vi "simx Get Objects.vi"(6 "operationMode":i32, 7 "objectHandles":i32, 8 "error in (no error)":errorcluster, 9 "objectCount":i32, 10 "objectType":i32, 11 "clientID":i32) -> (0 "error out":errorcluster, 1 "objectCount out":i32, 3 "function return":i32, 5 "objectHandles out":i32)   [LabVIEW 2019, in "PXL_V-REP.lvlib"]
doc: "EXTAPI_DLLEXPORT simxInt simxGetObjects(simxInt clientID,simxInt objectType,simxInt* objectCount,simxInt** objectHandles,simxInt operationMode);"
uses:
  PXL_V-REP.lvlib
  <userlib>/V-REP/remoteApi.dll
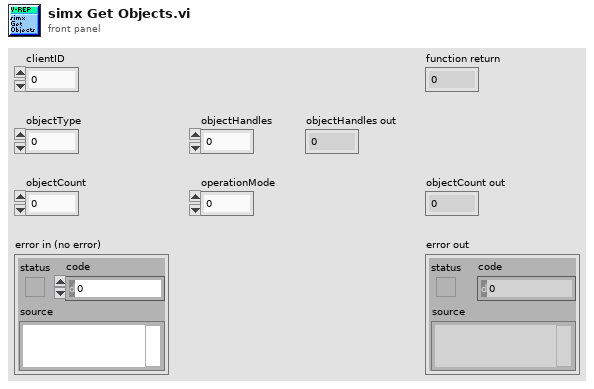
[diagram p1: front panel]
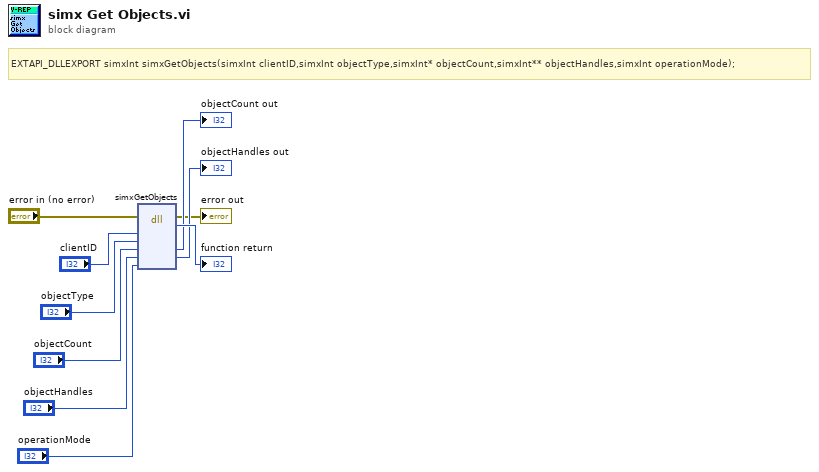
[diagram p0: block diagram]
diagram:
  # "EXTAPI_DLLEXPORT simxInt simxGetObjects(simxInt clientID,simxInt objectType,simxInt* objectCount,simxInt** objectHandles,simxInt operationMode);"
  n1 = dll-call lib="C:/Program Files (x86)/National Instruments/LabVIEW 2019/user.lib/V-REP/remoteApi.*" fn="simxGetObjects"(error in="error in (no error)", "clientID"="clientID", "objectType"="objectType", "objectCount"="objectCount", "objectHandles"="objectHandles", "operationMode"="operationMode") -> (error out=→"error out":errorcluster, →"function return":i32, "objectCount"=→"objectCount out":i32, "objectHandles"=→"objectHandles out":i32)  [unwired: 5 in, 1 out]
